vi "Configure.vi"(8 "error in (no error)":errorcluster, 11 "Common Measurements Interface in":refnum<class "Common Measurements Interface.lvclass">) -> (0 "error out":errorcluster, 3 "Common Measurements Interface out":refnum<class "Common Measurements Interface.lvclass">)   [LabVIEW 2015, in "Common Measurements Interface.lvclass"]
uses:
  Common Measurements Interface.lvclass
  Mag Lab Measure Interface/Mag Lab Measure UI.lvclass/Mag Lab Measure UI.ctl
  Common Measurements Interface.lvclass/Common Measurements Interface.ctl
  Queued Listbox/Queued Listbox.xctl
  Mag Lab Measure Interface/Interface with menu/Interface with menu.lvclass
  Mag Lab Measure Interface/Mag Lab Measure UI.lvclass
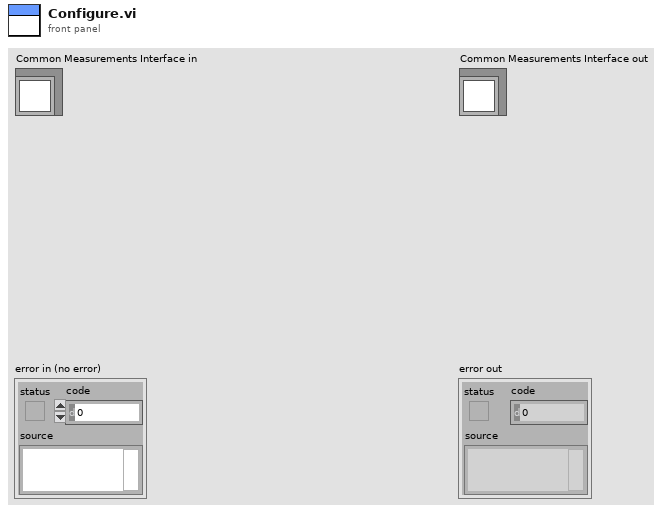
[diagram p1: front panel]
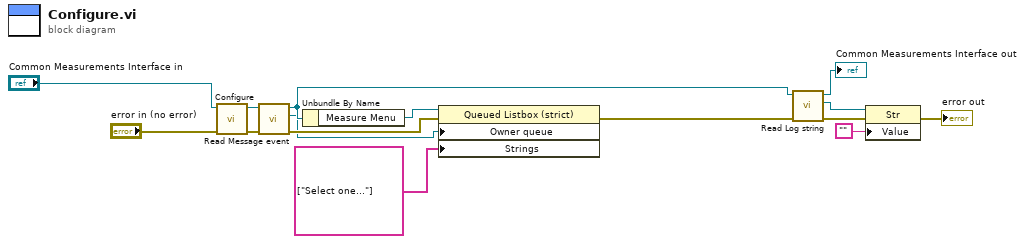
[diagram p0: block diagram]
diagram:
  n1 = call-parent "Configure.vi"("error in (no error)"="error in (no error)", "Mag Lab Measure Interface in"="Common Measurements Interface in") -> ("error out"=w13:errorcluster, "Mag Lab Measure Interface out"=w12:refnum<class "Common Measurements Interface.lvclass">)  [unwired: 8 in]
  n2 = call "Read Message event.vi"("error in (no error)"=w13, "Mag Lab Measure Interface in"=w12) -> ("error out"=w10:errorcluster, "Message event"=w3:refnum<user-event>, "Mag Lab Measure Interface out"=w9:refnum<class "Common Measurements Interface.lvclass">)  [unwired: 7 in]
  n3 = Unbundle By Name(w9) -> ("Measure Menu"=w11:refnum<vi>)
  n4 = property on="Property Node" class="Queued Listbox (strict)"(reference=w11, error in=w10, "Owner queue"=w3, "Strings"=string[] ["Select one..."] ("Menu object names")) -> (error out=w1:errorcluster)  [unwired: 1 out]
  n5 = call "Read Log string.vi"("error in (no error)"=w1, "Mag Lab Measure Interface in"=w9) -> ("error out"=w5:errorcluster, "Log string"=w6:refnum<vi>, "Mag Lab Measure Interface out"=→"Common Measurements Interface out":refnum<class "Common Measurements Interface.lvclass">)  [unwired: 7 in]
  n6 = property class="Str"(reference=w6, error in=w5, "Value"="") -> (error out=→"error out":errorcluster)  [unwired: 1 out]
